vi "000_Alin Manage.vi"(11 "Queue Ref In":T1={"UI"=refnum, "Message"=refnum, "Data"=refnum, "Caller"=refnum, "Name"="000 Common", "Data Path"=path "", "Class Path"=path "", "SubPanel"=refnum, "Project Name"="", "MNT"="", "Title"="", "Data Source"=refnum, "Queue List"={}, "VI"=refnum, "UE"=refnum}) -> ()   [LabVIEW 2020]
doc: "000001"
uses:
  Alin/QMH/000 Module Data Type.ctl
  Alin/QMH/Queue Message.ctl
panel:
  in  "AlinTree Refresh":bool
  in  "Exit Prepare":bool
  in  "Panel Show":bool
  in  "Data Source List":string(tree)
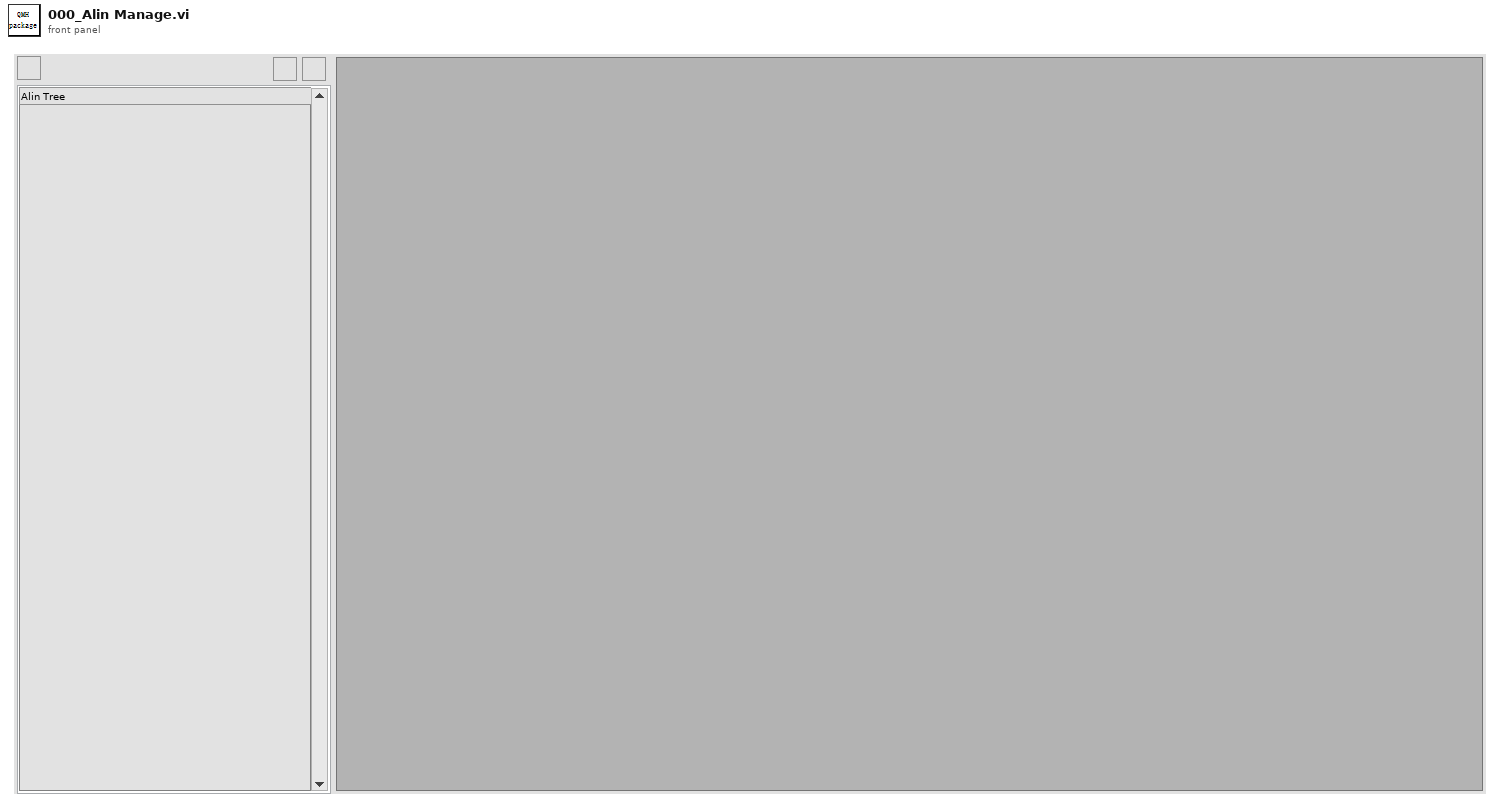
[diagram p1: front panel]
types:
  T1 = typedef "000 Module Data Type.ctl" = cluster{"UI":refnum<queue>, "Message":refnum<queue>, "Data":refnum<queue>, "Caller":refnum<queue>, "Name":string, "Data Path":path, "Class Path":path, "SubPanel":refnum<vi>, "Project Name":string, "MNT":string, "Title":string, "Data Source":refnum<queue>, "Queue List":map{string, refnum<queue>}, "VI":refnum<vi>, "UE":refnum<user-event>}
  T2 = cluster{"Queue":T1, "Delay":cluster{"Count Time(ms)":u32, "Delay Time(ms)":u32, "Next":string}, "SList":refnum<vi>}
  T3 = enum32{"Invalid", "Standard", "Closed", "Hidden", "Minimized", "Maximized"}
  T4 = cluster{"Caller":refnum<queue>, "Message":refnum<queue>}
  T5 = typedef "eventvkey.ctl" = enum16{"ASCII", "Enter", "Return", "Shift", "Ctrl", "Alt", "Cmd", "Opt", "Caps", "NumLock", "Clear", "Break", "Up", "Down", "Left", "Right", "Insert", "Delete", "Home", "End", "PageUp", "PageDown", "Escape", "Help", "Pause", "ScrollLock", "F1", "F2", "F3", "F4", "F5", "F6", "F7", "F8", "F9", "F10", "F11", "F12", "F13", "F14", "F15", "F16", "F17", "F18", "F19", "F20", "F21", "F22", "F23", "F24", "Play", "VolumeUp", "VolumeDown", "Mute", "Two Byte Char"}
  T6 = cluster{"Shift":bool, "Ctrl":bool, "Alt":bool, "Cmd":bool, "Opt":bool}
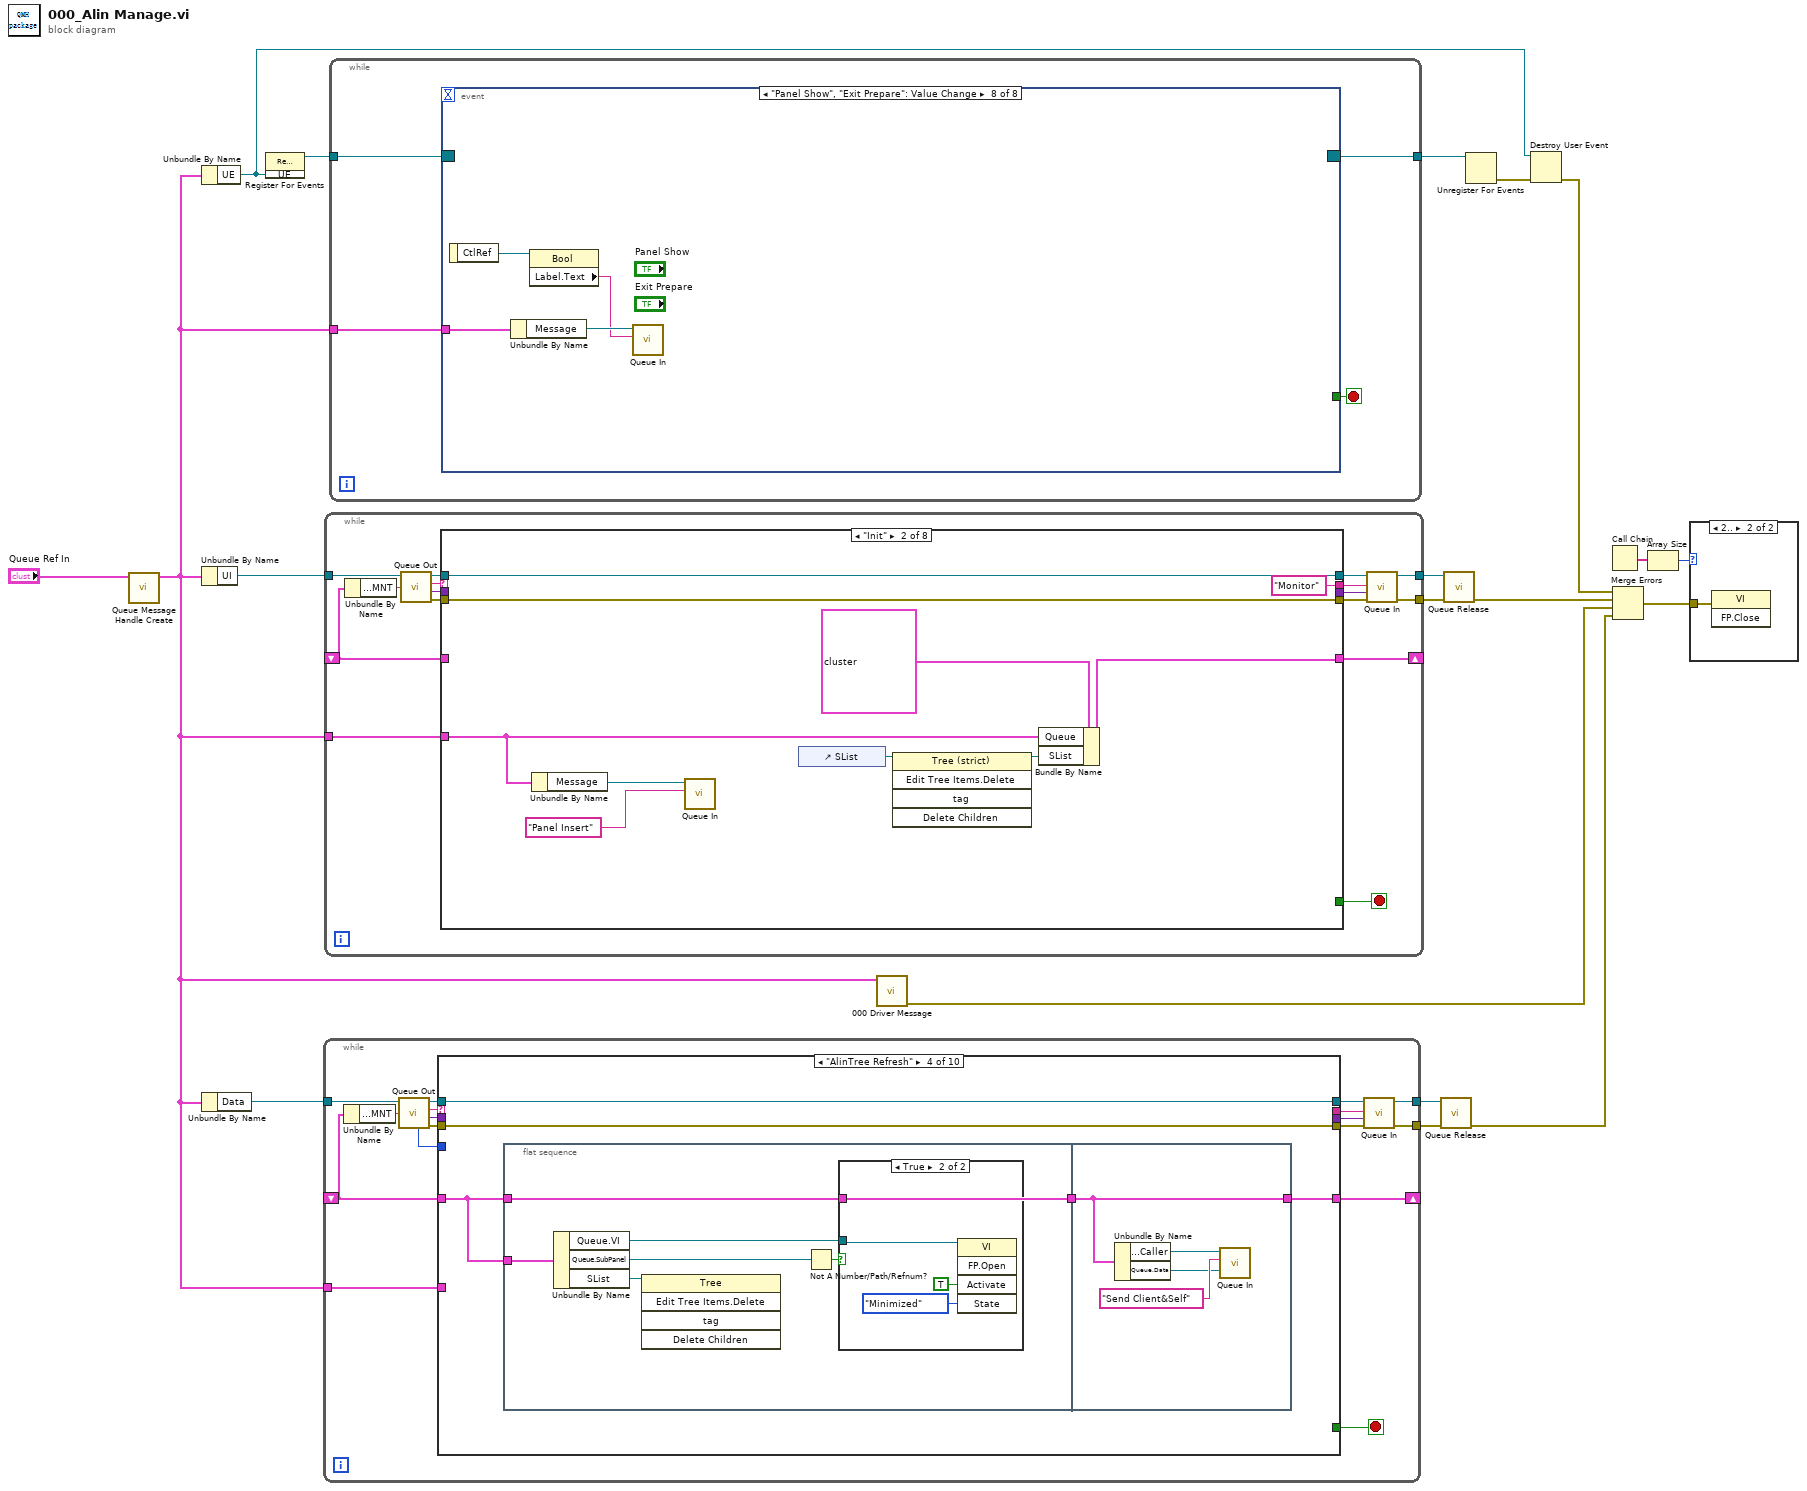
[diagram p0: block diagram]
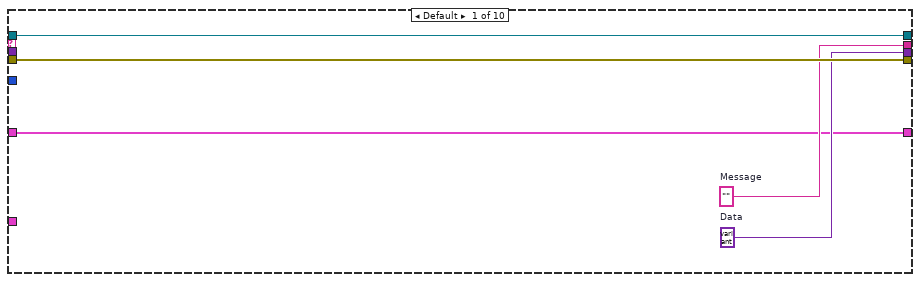
[diagram p2: hidden frame]
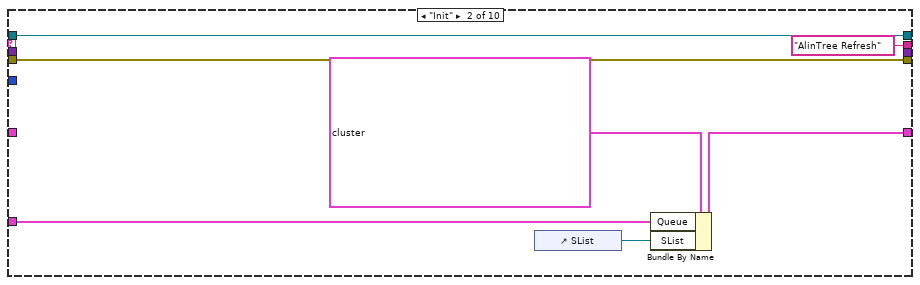
[diagram p3: hidden frame]
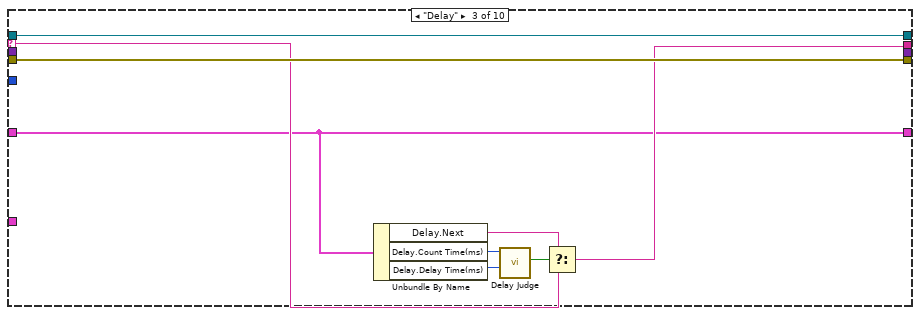
[diagram p4: hidden frame]
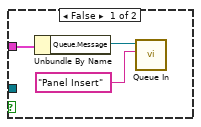
[diagram p5: hidden frame]
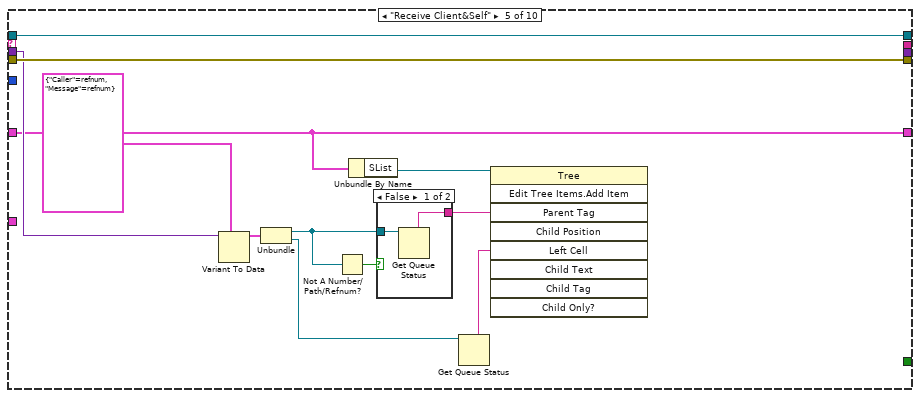
[diagram p6: hidden frame]
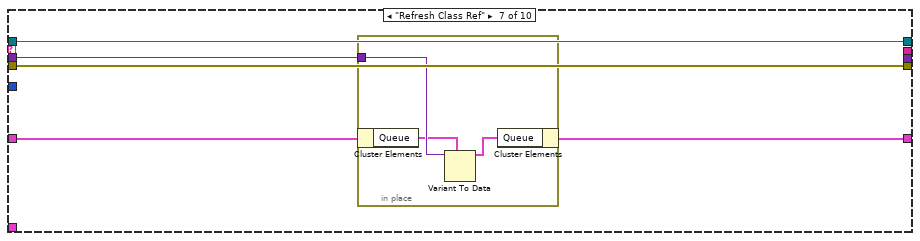
[diagram p9: hidden frame]
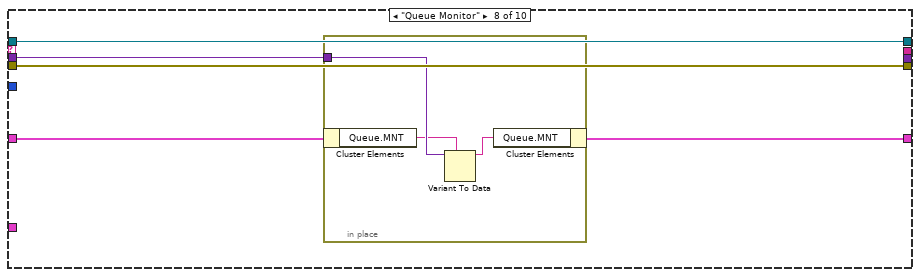
[diagram p10: hidden frame]
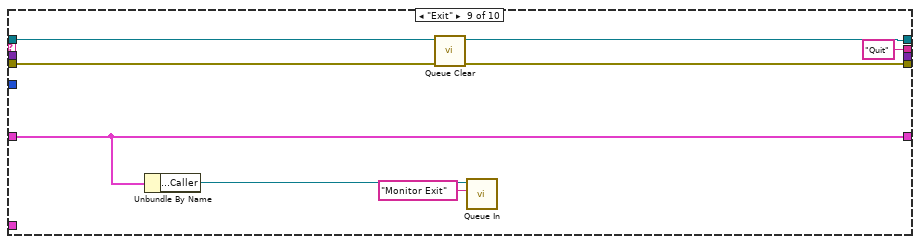
[diagram p11: hidden frame]
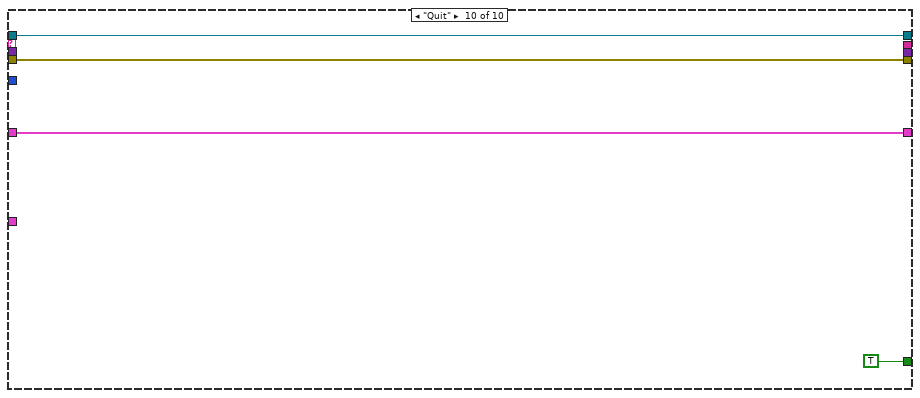
[diagram p12: hidden frame]
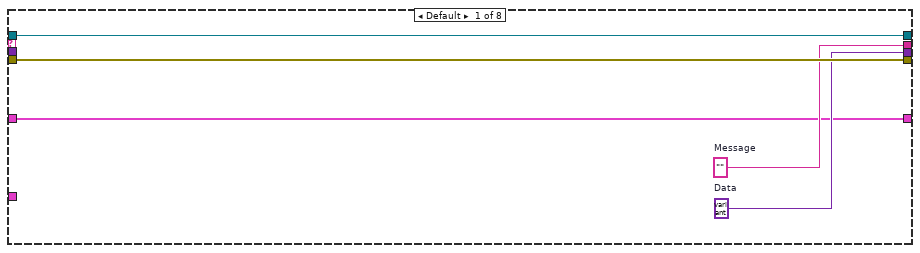
[diagram p14: hidden frame]
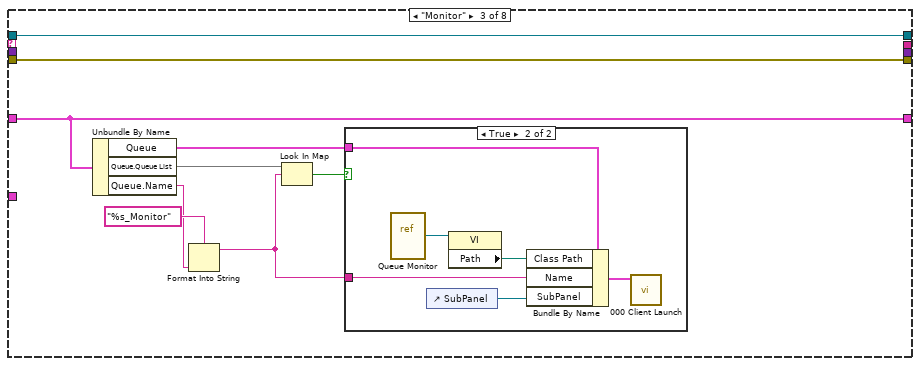
[diagram p15: hidden frame]
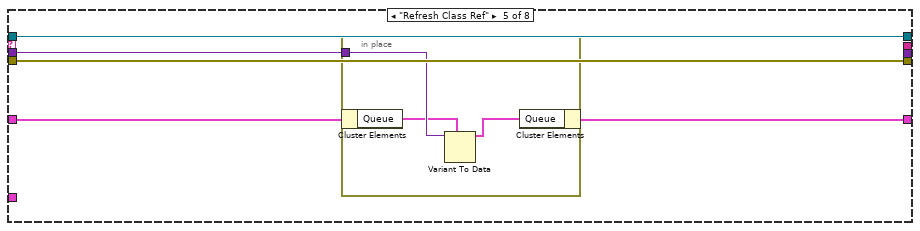
[diagram p18: hidden frame]
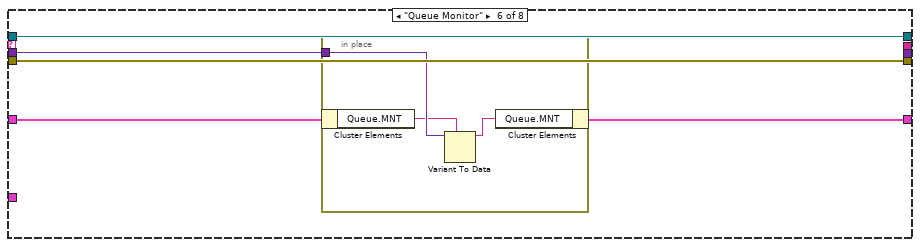
[diagram p19: hidden frame]
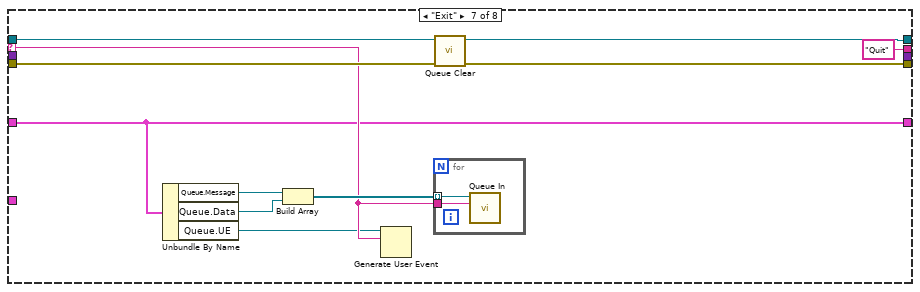
[diagram p20: hidden frame]
diagram:
  n1 = call "Queue Message Handle Create.vi"("Queue Ref In"="Queue Ref In") -> ("Queue Ref Out"=w1:T1)  [unwired: 8 in, 2 out]
  n2 = Unbundle By Name(w1) -> ("UE"=w3:refnum<user-event>)
  n3 = Unbundle By Name(w1) -> ("UI"=w14:refnum<queue>)
  n4 = Unbundle By Name(w1) -> ("Data"=w6:refnum<queue>)
  n5 = register-events(w3) -> (reference out=w19:refnum<event-registration>)  [unwired: 2 in, 1 out]
  n6 = while {
    tunnel: w6 -> [w32]
    tunnel: [w29] -> w8
    tunnel: [w28] -> w7
    shift-right: [w24] -> _
    shift-left: _ -> [w21]
    tunnel: w1 -> [w20]
    stop <- w36 stop-if-true
    n7 = Unbundle By Name(w21) -> ("Queue.MNT"=w22:string)
    n8 = call "Queue Out.vi"("Monitor"=w22, "Queue In"=w32) -> ("error out"=w35:errorcluster, "Data"=w33:variant, "Message"=w34:string, "Queue Out"=w31:refnum<queue>, "Queue NUmber"=w23:i32)  [unwired: 5 in]
    n9 = case shown="\"AlinTree Refresh\"" w34 {
      selector: w34 -> [_ _ w50 _ _ _ _ _ _ _]
      tunnel: w31 -> [w41 w48 w57 w61 w90 w95 w100 w108 w118 w122]
      tunnel: w35 -> [w40 w47 w56 w62 w89 w94 w99 w107 w116 w123]
      tunnel: [w41 w48 w57 w61 w90 w95 w100 w108 w117 w122] -> w30
      tunnel: [w40 w47 w56 w62 w89 w94 w99 w107 w115 w123] -> w27
      tunnel: [w39 "AlinTree Refresh" ("Next") w51 _ _ _ _ _ "Quit" _] -> w26
      tunnel: [_ _ _ _ _ _ _ _ _ TRUE] -> w36
      tunnel: [w38 _ _ _ _ _ _ _ _ _] -> w25
      tunnel: w33 -> [_ _ _ _ w88 _ w96 w104 _ _]
      tunnel: [w37 w44 w49 w58 w86 w93 w97 w105 w114 w120] -> w24
      tunnel: w21 -> [w37 _ w49 w60 w86 w93 w98 w106 w114 w120]
      tunnel: w23 -> [_ _ _ _ _ _ _ _ _ _]
      tunnel: w20 -> [_ w43 _ _ _ _ _ _ _ _]
      frame Default {
        w38 = variant  # Data
        w39 = ""  # Message
      }
      frame "Init" {
        n10 = control-ref of="SList"() -> (w42:refnum<vi>)
        n11 = Bundle By Name(cluster=T2 {"Queue"={"UI"=refnum, "Message"=refnum, "Data"=refnum, "Caller"=refnum, "Name"="000 Common", "Data Path"=path "", "Class Path"=path "", "SubPanel"=refnum, "Project Name"="", "MNT"="", "Title"="", "Data Source"=refnum, "Queue List"={}, "VI"=refnum, "UE"=refnum}, "Delay"={"Count Time(ms)"=250, "Delay Time(ms)"=250, "Next"="Receive Data,Delay"}, "SList"=refnum}, "Queue"=w43, "SList"=w42) -> (w44:T2)
      }
      frame "Delay" {
        n12 = Unbundle By Name(w49) -> ("Delay.Next"=w55:string, "Delay.Count Time(ms)"=w52:u32, "Delay.Delay Time(ms)"=w53:u32)
        n13 = call "Delay Judge.vi"("Delay Time(ms)"=w53, "Count Time(ms)"=w52) -> ("Time Out?"=w54:bool)  [unwired: 5 in, 4 out]
        n14 = Select(t=w55, s=w54, f=w50) -> (s? t:f=w51:string)
      }
      frame "AlinTree Refresh" {
        n15 = flat-sequence {
          tunnel: w60 -> [w68]
          tunnel: w60 -> [w63]
          tunnel: [w63] -> w59
          tunnel: w59 -> [w76]
          tunnel: [w76] -> w58
          frame #0 {
            n16 = Unbundle By Name(w68) -> ("Queue.VI"=w64:refnum<vi>, "Queue.SubPanel"=w65:refnum<vi>, "SList"=w67:refnum<vi>)
            n17 = invoke class="Tree" method="Edit Tree Items.Delete"(reference=w67) -> ()  [unwired: 4 in, 5 out]
            n18 = Not A Number/Path/Refnum?(number/path/refnum=w65) -> (NaN/Path/Refnum?=w66:bool)
            n19 = case shown="True" w66 {
              tunnel: w64 -> [_ w74]
              tunnel: w63 -> [w71 _]
              frame False {
                n20 = Unbundle By Name(w71) -> ("Queue.Message"=w70:refnum<queue>)
                n21 = call "Queue In.vi"("Message"="Panel Insert", "Queue In"=w70) -> ()  [unwired: 8 in, 2 out]
              }
              frame True {
                n22 = invoke class="VI" method="FP.Open"(reference=w74, "Activate"=TRUE ("激活？"), "State"=T3."Minimized" ("状态")) -> ()  [unwired: 2 in, 5 out]
              }
            }
          }
          frame #1 {
            n23 = Unbundle By Name(w76) -> ("Queue.Caller"=w78:refnum<queue>, "Queue.Data"=w75:refnum<queue>)
            n24 = call "Queue In.vi"("Data"=w75, "Message"="Send Client&Self", "Queue In"=w78) -> ()  [unwired: 7 in, 2 out]
          }
        }
      }
      frame "Receive Client&Self" {
        n25 = Variant To Data(type=T4 {"Caller"=refnum, "Message"=refnum} ("输出簇"), Variant=w88) -> (data=w85:T4)  [unwired: 1 in, 1 out]
        n26 = Unbundle(w85) -> ("Caller"=w82:refnum<queue>, "Message"=w80:refnum<queue>)
        n27 = Not A Number/Path/Refnum?(number/path/refnum=w82) -> (NaN/Path/Refnum?=w83:bool)
        n28 = Unbundle By Name(w86) -> ("SList"=w84:refnum<vi>)
        n29 = case shown="False" w83 {
          tunnel: w82 -> [w92 _]
          tunnel: [w91 _] -> w81
          frame False {
            n30 = Get Queue Status(queue=w92) -> (queue name=w91:string)  [unwired: 2 in, 7 out]
          }
          frame True {
          }
        }
        n31 = Get Queue Status(queue=w80) -> (queue name=w79:string)  [unwired: 2 in, 7 out]
        n32 = invoke class="Tree" method="Edit Tree Items.Add Item"(reference=w84, "Parent Tag"=w81, "Left Cell"=w79) -> ()  [unwired: 6 in, 9 out]
      }
      frame "====System====" {
      }
      frame "Refresh Class Ref" {
        n33 = in-place {
          in-place-border: w96 -> [w103]
          n34 = in-place-cluster #1(w98) -> ("Queue"=w102:T1)
          n35 = Variant To Data(type=w102, Variant=w103) -> (data=w101:T1)  [unwired: 1 in, 1 out]
          n36 = in-place-cluster #1("Queue"=w101) -> (w97:T2)
        }
      }
      frame "Queue Monitor" {
        n37 = in-place {
          in-place-border: w104 -> [w111]
          n38 = in-place-cluster #2(w106) -> ("Queue.MNT"=w110:string)
          n39 = Variant To Data(type=w110, Variant=w111) -> (data=w109:string)  [unwired: 1 in, 1 out]
          n40 = in-place-cluster #2("Queue.MNT"=w109) -> (w105:T2)
        }
      }
      frame "Exit" {
        n41 = Unbundle By Name(w114) -> ("Queue.Caller"=w113:refnum<queue>)
        n42 = call "Queue Clear.vi"("error in (no error)"=w116, "Queue In"=w118) -> ("error out"=w115:errorcluster, "Queue Out"=w117:refnum<queue>)  [unwired: 8 in]
        n43 = call "Queue In.vi"("Message"="Monitor Exit", "Queue In"=w113) -> ()  [unwired: 8 in, 2 out]
      }
      frame "Quit" {
      }
    }
    n44 = call "Queue In.vi"("error in (no error)"=w27, "Data"=w25, "Message"=w26, "Queue In"=w30) -> ("error out"=w28:errorcluster, "Queue Out"=w29:refnum<queue>)  [unwired: 6 in]
  }
  n45 = while {
    tunnel: w14 -> [w135]
    tunnel: [w132] -> w16
    tunnel: [w131] -> w15
    shift-right: [w127] -> _
    shift-left: _ -> [w126]
    tunnel: w1 -> [w124]
    stop <- w139 stop-if-true
    n46 = Unbundle By Name(w126) -> ("Queue.MNT"=w125:string)
    n47 = call "Queue Out.vi"("Monitor"=w125, "Queue In"=w135) -> ("error out"=w138:errorcluster, "Data"=w136:variant, "Message"=w137:string, "Queue Out"=w134:refnum<queue>)  [unwired: 5 in, 1 out]
    n48 = case shown="\"Init\"" w137 {
      selector: w137 -> [_ _ _ _ _ _ w191 _]
      tunnel: w134 -> [w144 w154 w163 w172 w177 w185 w198 w204]
      tunnel: w138 -> [w143 w153 w162 w171 w176 w184 w196 w205]
      tunnel: [w144 w154 w163 w172 w177 w185 w197 w204] -> w133
      tunnel: [w143 w153 w162 w171 w176 w184 w195 w205] -> w130
      tunnel: [w142 "Monitor" ("Message") _ _ _ _ "Quit" _] -> w129
      tunnel: [_ _ _ _ _ _ _ TRUE] -> w139
      tunnel: [w141 _ _ _ _ _ _ _] -> w128
      tunnel: w136 -> [_ _ _ _ w173 w181 _ _]
      tunnel: [w140 w151 w161 w170 w174 w182 w190 w202] -> w127
      tunnel: w126 -> [w140 _ w161 w170 w175 w183 w190 w202]
      tunnel: w124 -> [_ w147 _ _ _ _ _ _]
      frame Default {
        w141 = variant  # Data
        w142 = ""  # Message
      }
      frame "Init" {
        n49 = Unbundle By Name(w147) -> ("Message"=w146:refnum<queue>)
        n50 = call "Queue In.vi"("Message"="Panel Insert", "Queue In"=w146) -> ()  [unwired: 8 in, 2 out]
        n51 = control-ref of="SList"() -> (w150:refnum<vi>)
        n52 = invoke class="Tree (strict)" method="Edit Tree Items.Delete"(reference=w150) -> (reference out=w149:refnum<vi>)  [unwired: 4 in, 4 out]
        n53 = Bundle By Name(cluster=cluster{"Queue":T1, "SList":refnum<vi>} {"Queue"={"UI"=refnum, "Message"=refnum, "Data"=refnum, "Caller"=refnum, "Name"="000 Common", "Data Path"=path "", "Class Path"=path "", "SubPanel"=refnum, "Project Name"="", "MNT"="", "Title"="", "Data Source"=refnum, "Queue List"={}, "VI"=refnum, "UE"=refnum}, "SList"=refnum}, "Queue"=w147, "SList"=w149) -> (w151:cluster{"Queue":T1, "SList":refnum<vi>})
      }
      frame "Monitor" {
        n54 = Unbundle By Name(w161) -> ("Queue"=w155:T1, "Queue.Queue List"=w160:map{string, refnum<queue>}, "Queue.Name"=w158:string)
        n55 = Format Into String(format string="%s_Monitor" ("格式字符串"), w158) -> (resulting string=w156:string)  [unwired: 2 in, 1 out]
        n56 = Look In Map(map=w160, key=w156) -> (key not found?=w157:bool)  [unwired: 1 in, 1 out]
        n57 = case shown="True" w157 {
          tunnel: w156 -> [_ w166]
          tunnel: w155 -> [_ w165]
          frame False {
          }
          frame True {
            n58 = vi-ref "Queue Monitor.vi"() -> (w169:refnum<vi>)
            n59 = control-ref of="SubPanel"() -> (w164:refnum<vi>)
            n60 = property class="VI"(reference=w169) -> ("Path"=w168:path)  [unwired: 1 in, 2 out]
            n61 = Bundle By Name(cluster=w165, "Class Path"=w168, "Name"=w166, "SubPanel"=w164) -> (w167:T1)
            n62 = call "000 Client Launch.vi"("Queue Ref"=w167) -> ()  [unwired: 10 in, 1 out]
          }
        }
      }
      frame "====System====" {
      }
      frame "Refresh Class Ref" {
        n63 = in-place {
          in-place-border: w173 -> [w180]
          n64 = in-place-cluster #3(w175) -> ("Queue"=w179:T1)
          n65 = Variant To Data(type=w179, Variant=w180) -> (data=w178:T1)  [unwired: 1 in, 1 out]
          n66 = in-place-cluster #3("Queue"=w178) -> (w174:cluster{"Queue":T1, "SList":refnum<vi>})
        }
      }
      frame "Queue Monitor" {
        n67 = in-place {
          in-place-border: w181 -> [w188]
          n68 = in-place-cluster #4(w183) -> ("Queue.MNT"=w187:string)
          n69 = Variant To Data(type=w187, Variant=w188) -> (data=w186:string)  [unwired: 1 in, 1 out]
          n70 = in-place-cluster #4("Queue.MNT"=w186) -> (w182:cluster{"Queue":T1, "SList":refnum<vi>})
        }
      }
      frame "Exit" {
        n71 = Unbundle By Name(w190) -> ("Queue.Message"=w194:refnum<queue>, "Queue.Data"=w193:refnum<queue>, "Queue.UE"=w189:refnum<user-event>)
        n72 = Build Array(w194, w193) -> (w192:refnum<queue>[])
        n73 = Generate User Event(user event=w189, event data cluster=w191) -> ()  [unwired: 2 in, 2 out]
        n74 = for {
          tunnel: w192 -> [w201] mode=indexing
          tunnel: w191 -> [w200]
          n75 = call "Queue In.vi"("Message"=w200, "Queue In"=w201) -> ()  [unwired: 8 in, 2 out]
        }
        n76 = call "Queue Clear.vi"("error in (no error)"=w196, "Queue In"=w198) -> ("error out"=w195:errorcluster, "Queue Out"=w197:refnum<queue>)  [unwired: 8 in]
      }
      frame "Quit" {
      }
    }
    n77 = call "Queue In.vi"("error in (no error)"=w130, "Data"=w128, "Message"=w129, "Queue In"=w133) -> ("error out"=w131:errorcluster, "Queue Out"=w132:refnum<queue>)  [unwired: 6 in]
  }
  n78 = while {
    tunnel: w19 -> [w209]
    tunnel: [w207] -> w18
    tunnel: w1 -> [w206]
    stop <- w208 stop-if-true
    n79 = event shown="[7] \"Panel Show\", \"Exit Prepare\": Value Change" {
      selector: w209 -> [_ _ _ _ _ _ _ _]
      dyn-events: [_ _ _ _ _ _ _ _] -> w207
      timeout: _ -> [_ _ _ _ _ _ _ _]
      tunnel: [_ _ _ _ w232 _ _ _] -> w208
      tunnel: w206 -> [_ w210 w217 w222 _ w237 _ w246]
      event Timeout {
        n80 = event-data() -> ()  [unwired: 1 in, 1 out]
      }
      event Key Down {
        n81 = event-data() -> ("Char"=w214:i16, "VKey"=w213:T5, "Mods"=w212:cluster{"Num Pad":bool, "Menu Key":bool}, "PlatMods"=w211:T6)  [unwired: 1 in]
        n82 = call "Queue Key Down.vi"("Queue Ref Out"=w210, "C"=w214, "Platform Key"=w211, "Group Key"=w212, "V Key"=w213) -> ()  [unwired: 6 in, 1 out]
      }
      event "AlinTree Refresh": Value Change {
        n83 = event-data() -> ("CtlRef"=w218:refnum<vi>)  [unwired: 1 in]
        n84 = Unbundle By Name(w217) -> ("Data"=w216:refnum<queue>)
        n85 = property class="Bool"(reference=w218) -> ("Label.Text"=w215:string)  [unwired: 1 in, 2 out]
        n86 = call "Queue In.vi"("Message"=w215, "Queue In"=w216) -> ()  [unwired: 8 in, 2 out]
      }
      event "Data Source List": Shortcut Menu Selection (User) {
        n87 = event-data() -> ("CtlRef"=w224:refnum<vi>, "ItemTag"=w225:string)  [unwired: 1 in]
        n88 = property class="Tree (strict)"(reference=w224) -> ("Value"=w223:string)  [unwired: 1 in, 2 out]
        n89 = case shown="Default" w223 {
          selector: w223 -> [w231 _]
          tunnel: w225 -> [w229 _]
          tunnel: [w230 _] -> w220
          tunnel: [w229 _] -> w219
          frame Default {
            n90 = call "Queue Send Message.vi"("Message"=w229, "Queue Name"=w231) -> ("error out"=w230:errorcluster)  [unwired: 7 in, 2 out]
          }
          frame "" {
          }
        }
        n91 = Unbundle By Name(w222) -> ("Data"=w221:refnum<queue>)
        n92 = case shown="\"Exit Prepare\"" w219 {
          tunnel: w221 -> [_ w228]
          tunnel: w220 -> [_ w226]
          frame "假", Default {
          }
          frame "Exit Prepare" {
            n93 = call "Queue In.vi"("error in (no error)"=w226, "Message"="AlinTree Refresh", "Queue In"=w228) -> ()  [unwired: 7 in, 2 out]
          }
        }
      }
      event User Event {
        n94 = event-data() -> ("Message"=w234:string)  [unwired: 1 in]
        n95 = Equal?(x=w234, y="Exit") -> (x = y?=w232:bool)
      }
      event Panel Close? {
        n96 = event-data() -> ()  [unwired: 1 in, 1 out]
        n97 = Unbundle By Name(w237) -> ("Message"=w236:refnum<queue>)
        n98 = call "Queue In.vi"("Message"="Exit Prepare", "Queue In"=w236) -> ()  [unwired: 8 in, 2 out]
        n99 = event-data("Discard?"=TRUE ("放弃？")) -> ()  [unwired: 1 in, 1 out]
      }
      event "Data Source List": Double Click {
        n100 = event-data() -> ("CtlRef"=w239:refnum<vi>)  [unwired: 1 in]
        n101 = property class="Tree (strict)"(reference=w239) -> ("Value"=w240:string)  [unwired: 1 in, 2 out]
        n102 = case shown="Default" w240 {
          selector: w240 -> [w242 _]
          frame Default {
            n103 = call "Queue Send Message.vi"("Message"="Panel Show", "Queue Name"=w242) -> ()  [unwired: 7 in, 3 out]
          }
          frame "" {
          }
        }
      }
      event "Panel Show", "Exit Prepare": Value Change {
        n104 = event-data() -> ("CtlRef"=w244:refnum<vi>)  [unwired: 1 in]
        n105 = Unbundle By Name(w246) -> ("Message"=w245:refnum<queue>)
        n106 = property class="Bool"(reference=w244) -> ("Label.Text"=w243:string)  [unwired: 1 in, 2 out]
        n107 = call "Queue In.vi"("Message"=w243, "Queue In"=w245) -> ()  [unwired: 8 in, 2 out]
      }
    }
  }
  n108 = call "000 Driver Message.vi"("Queue In"=w1) -> ("error out"=w4:errorcluster)  [unwired: 8 in, 2 out]
  n109 = call "Queue Release.vi"("error in (no error)"=w7, "Queue In"=w8) -> ("error out"=w5:errorcluster)  [unwired: 9 in]
  n110 = call "Queue Release.vi"("error in (no error)"=w15, "Queue In"=w16) -> ("error out"=w12:errorcluster)  [unwired: 9 in]
  n111 = Unregister For Events(event registration refnum=w18) -> (error out=w17:errorcluster)  [unwired: 1 in]
  n112 = Destroy User Event(user event=w3, error in=w17) -> (error out=w13:errorcluster)
  n113 = Call Chain() -> (call chain=w10:string[])
  n114 = Merge Errors(w13, w12, w4, w5) -> (w11:errorcluster)
  n115 = Array Size(array=w10) -> (size(s)=w9:i32)
  n116 = case shown="2.." w9 {
    tunnel: w11 -> [_ w247]
    frame 0, Default {
    }
    frame 2.. {
      n117 = invoke class="VI" method="FP.Close"(error in=w247) -> ()  [unwired: 2 in, 3 out]
    }
  }
